vi "fftw_memcpy_from_real_dbl.vi"(8 "error in (no error)":errorcluster, 10 "source dbl array":dbl[](array[numeric]), 11 "*data_out":u64) -> (0 "error out":errorcluster, 3 "*data_out (copy)":u64)   [LabVIEW 2020, in "FFTWDLL.lvlib"]
doc: "Copy source double array to FFTW array."
uses:
  FFTWDLL.lvlib
  ntdll.dll
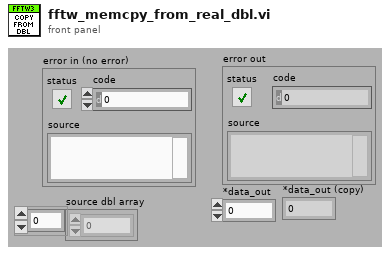
[diagram p1: front panel]
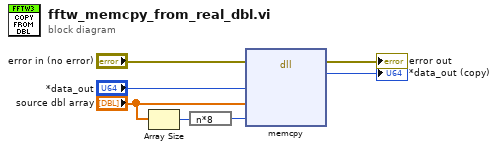
[diagram p0: block diagram]
diagram:
  n1 = Array Size(array="source dbl array") -> (size(s)=w4:i32)
  n2 = expression code="n*8"(w4) -> (w3:i32)
  n3 = dll-call lib="ntdll.dll" fn="memcpy"(error in="error in (no error)", "dest"="*data_out", "src"="source dbl array", "n"=w3) -> (error out=→"error out":errorcluster, "dest"=→"*data_out (copy)":u64)  [unwired: 5 in, 1 out]
